vi "Initialize-object-wrapper-example.vi"(8 "error in (no error)":errorcluster) -> (0 "error out":errorcluster, 3 "SM1000-control out":T1)   [LabVIEW 2013, in "MaterialCharacterization.lvlib" / "MC-SM1000.lvclass"]
uses:
  MC-SM1000.lvclass
  Object-reference.ctl
  TCP-settings.ctl
  DOTNET-settings.ctl
  Device-identification.ctl
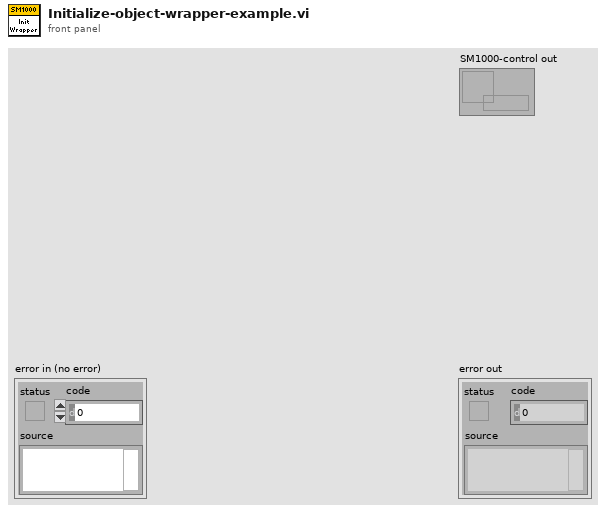
[diagram p1: front panel]
types:
  T1 = typedef "MaterialCharacterization.lvlib/MC-SM1000.lvclass/Object-reference.ctl" = refnum<data-value>
  T2 = typedef "MaterialCharacterization.lvlib/MC-SM1000.lvclass/DOTNET-settings.ctl" = cluster{"Target IP":string, "Target broadcast port":i32, "Target communication port":i32, "clientID":i32, "Broadcast IP":string, "Servercount":i32, "Device IDs":T3[]}
  T3 = typedef "MaterialCharacterization.lvlib/MC-SM1000.lvclass/Device-identification.ctl" = cluster{"Name":string, "IP":string, "Mac address":string}
  T4 = typedef "MaterialCharacterization.lvlib/MC-SM1000.lvclass/TCP-settings.ctl" = cluster{"Target IP":string, "Target TCP port":u16, "TCP read mode":enum16{"Standard", "Buffered", "CRLF", "Immediate"}, "TCP read buffer":i32, "Read timeout":i32}
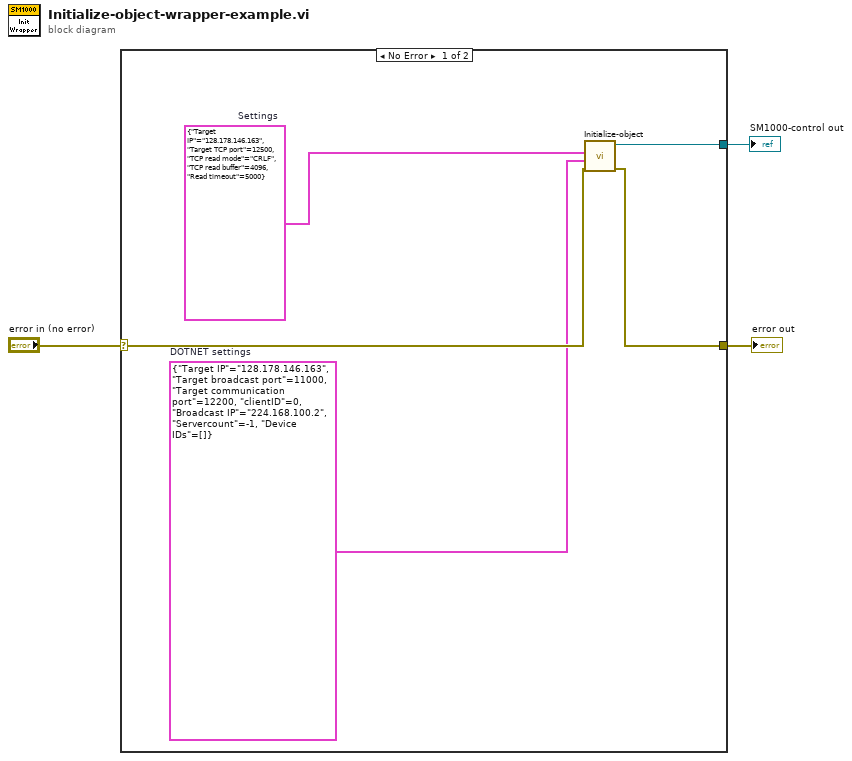
[diagram p0: block diagram]
diagram:
  n1 = case shown="No Error" "error in (no error)" {
    selector: "error in (no error)" -> [w7 w9]
    tunnel: [w6 w9] -> w2
    tunnel: [w8 _] -> w1
    frame No Error {
      w4 = T2 {"Target IP"="128.178.146.163", "Target broadcast port"=11000, "Target communication port"=12200, "clientID"=0, "Broadcast IP"="224.168.100.2", "Servercount"=-1, "Device IDs"=[]}  # DOTNET settings
      w5 = T4 {"Target IP"="128.178.146.163", "Target TCP port"=12500, "TCP read mode"=enum."CRLF", "TCP read buffer"=4096, "Read timeout"=5000}  # Settings
      n2 = call "Initialize-object.vi"("error in (no error)"=w7, "DOTNET settings"=w4, "TCP settings"=w5) -> ("error out"=w6:errorcluster, "SM1000-control out"=w8:T1)  [unwired: 7 in]
    }
    frame Error {
    }
  }
  "error out" <- w2
  "SM1000-control out" <- w1
